vi "Alternate BG Color.vi"(7 "Number of Rows":i32, 8 "错误输入":errorcluster, 9 "Second BG Color":u32(colorbox), 10 "First BG Color":u32(colorbox), 11 "Listbox Ref":refnum<vi>) -> (0 "错误输出":errorcluster, 3 "Dup Listbox Ref":refnum<vi>)   [LabVIEW 2012, in "Listbox Tool.lvlib"]
uses:
  Listbox Tool.lvlib
  Property/Set and Get Active Row BG Color.vi
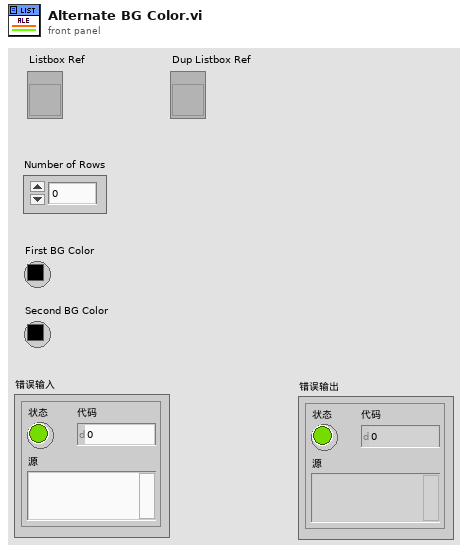
[diagram p1: front panel]
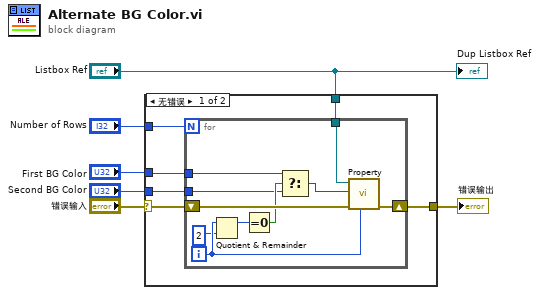
[diagram p0: block diagram]
diagram:
  n1 = case shown="无错误" "错误输入" {
    selector: "错误输入" -> [w12 w23]
    tunnel: [w11 w23] -> w5
    tunnel: "Number of Rows" -> [w10 _]
    tunnel: "First BG Color" -> [w9 _]
    tunnel: "Second BG Color" -> [w8 _]
    tunnel: "Listbox Ref" -> [w7 _]
    frame No Error {
      n2 = for {
        N: w10 -> [_]
        shift-right: [w21] -> w11
        shift-left: w12 -> [w22]
        tunnel: w9 -> [w16]
        tunnel: w8 -> [w15]
        tunnel: w7 -> [w14]
        i -> [w20]
        n3 = Quotient & Remainder(x=w20, y=2) -> (x-y*floor(x/y)=w18:i32)  [unwired: 1 out]
        n4 = Equal To 0?(x=w18) -> (x = 0?=w17:bool)
        n5 = Select(t=w16, s=w17, f=w15) -> (s? t:f=w13:u32)
        n6 = call-poly "Property.vi"("Active Row"=w20, "错误输入"=w22, "CellBG In"=w13, "Listbox Ref"=w14) -> ("错误输出"=w21:errorcluster)  [unwired: 5 in, 2 out]
      }
    }
    frame Error {
    }
  }
  "错误输出" <- w5
  "Dup Listbox Ref" <- "Listbox Ref"
